vi "GUI.vi"() -> ()   [LabVIEW 2014]
uses:
  <vilib>/Platform/TimedLoop/XDataNode/timing_clust.ctl
  <vilib>/Platform/TimedLoop/XDataNode/nitl_modes.ctl
  <vilib>/Platform/TimedLoop/XDataNode/wakeup.ctl
  <vilib>/Instr/_visa.llb/VISA Configure Serial Port (Instr).vi
  <vilib>/platform/TimedLoop/XDataNode/XDataNode.xnode
  <vilib>/Platform/TimedLoop/XDataNode/XDNodeRunTimeDep.lvlib
panel:
  out "password is wrong":bool
  in  "write buffer":string
  in  "Write":bool
  in  "byte count":u32
  out "return count read":u32
  out "return count write":u32
  out "read buffer":string
  in  "Read":bool
  in  "timeout (10sec)":u32=10000
  in  "VISA resource name":refnum<visa-resource-name>
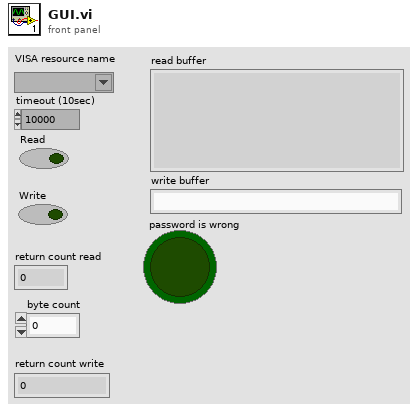
[diagram p1: front panel]
types:
  T1 = typedef "XDNodeRunTimeDep.lvlib/timing_clust.ctl" = cluster{"Expected End [f-1]":u64, "Actual End [f-1]":u64, "Finished Late? [f-1]":bool, "Expected End [i-1]":u64, "Actual End [i-1]":u64, "Finished Late? [i-1]":bool, "Expected Start [i]":u64, "Actual Start [i]":u64, "Expected Start [f]":u64, "Actual Start [f]":u64, "Source Name":string, "Structure Name":string, "Period":i64, "Deadline":i64, "Offset":i64, "Start":i64, "Priority":i32, "Timeout":i32, "Mode":T2, "Wakeup Reason":T3, "Error":errorcluster, "Source Type":string, "Secondary Source Type":string, "Global End Time":u64, "Global Start Time":u64, "Frame Duration":u64, "Iteration Duration":u64, "Assigned CPU":i32, "I/O Scan Engine Mode":u32}
  T2 = typedef "XDNodeRunTimeDep.lvlib/nitl_modes.ctl" = enum32{"No Change", "Process missed periods, maintain original phase", "Discard missed periods, maintain original phase", "Process missed periods, ignore original phase", "Discard missed periods, ignore original phase"}
  T3 = typedef "XDNodeRunTimeDep.lvlib/wakeup.ctl" = enum32{"Normal", "Aborted", "Asynchronous wakeup", "Timing source error", "Timed loop error", "Timeout"}
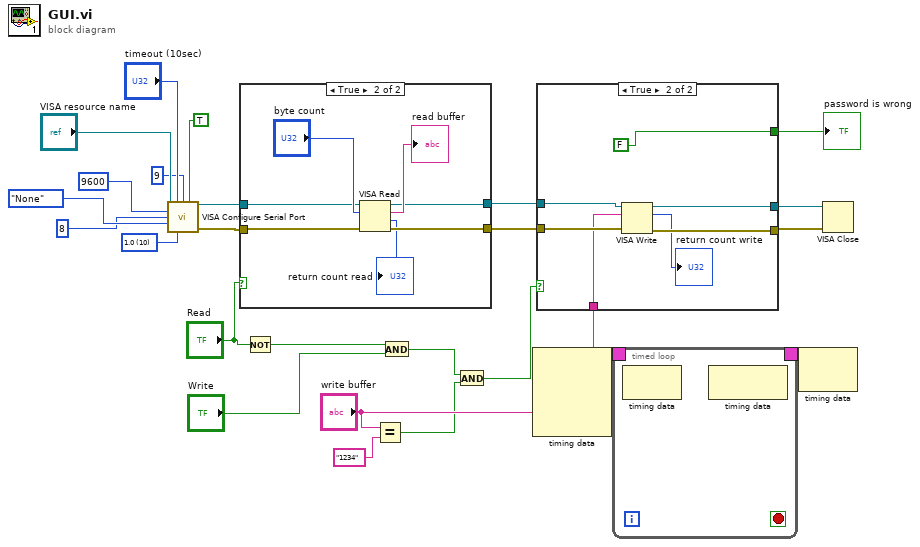
[diagram p0: block diagram]
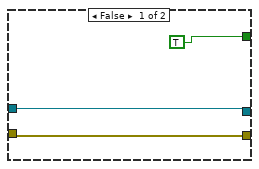
[diagram p3: hidden frame]
diagram:
  w22 = u16 10 items=["1.0"=10, "1.5"=15, "2.0"=20] ("stop bits (10: 1 bit)")
  n1 = call-poly "VISA Configure Serial Port"("VISA resource name"="VISA resource name", "timeout (10sec)"="timeout (10sec)", "termination char\n(0xA = '\\n' = LF)"=u8 9 ("termination char\n(0xA = '\\n' = LF)"), "Enable Termination\nChar (T)"=TRUE ("Enable Termination\nChar (T)"), "baud rate (9600)"=u32 9600, "data bits (8)"=u16 8, "parity (0:none)"=enum16{"None", "Odd", "Even", "Mark", "Space"}."None", "stop bits (10: 1 bit)"=w22) -> ("VISA resource name out"=w13:refnum<visa-resource-name>, "error out"=w11:errorcluster)  [unwired: 6 in]
  n2 = case shown="True" "Read" {
    tunnel: w11 -> [w27 w31]
    tunnel: [w26 w28] -> w12
    tunnel: [w27 w34] -> w10
    tunnel: w13 -> [w26 w29]
    frame False {
    }
    frame True {
      n3 = VISA Read(VISA resource name=w29, byte count="byte count", error in (no error)=w31) -> (VISA resource name out=w28:refnum<visa-resource-name>, read buffer=→"read buffer":string, return count=→"return count read":u32, error out=w34:errorcluster)
    }
  }
  n4 = Not(x="Read") -> (.not. x?=w16:bool)
  n5 = Equal?(x="write buffer", y="1234") -> (x = y?=w4:bool)
  n6 = And(x=w16, y="Write") -> (x .and. y?=w8:bool)
  n7 = And(x=w8, y=w4) -> (x .and. y?=w7:bool)
  n8 = node-c288() -> (w2:T1)  [unwired: 4 in]
  n9 = case shown="True" w7 {
    tunnel: w10 -> [w37 w44]
    tunnel: [w36 w43] -> w18
    tunnel: [w37 w42] -> w17
    tunnel: w12 -> [w36 w40]
    tunnel: "write buffer" -> [_ w39]
    tunnel: [TRUE FALSE] -> w5
    frame False {
    }
    frame True {
      n10 = VISA Write(VISA resource name=w40, write buffer=w39, error in (no error)=w44) -> (VISA resource name out=w43:refnum<visa-resource-name>, return count=→"return count write":u32, error out=w42:errorcluster)
    }
  }
  "password is wrong" <- w5
  n11 = timed-loop {
    timing: w2 -> [_]
    timing-out: [_] -> w1
    stop <- _ stop-if-true
    n12 = node-c288() -> ()  [unwired: 1 in, 1 out]
    n13 = node-c288() -> ()  [unwired: 1 in, 1 out]
  }
  n14 = node-c288(w1) -> ()  [unwired: 1 out]
  n15 = VISA Close(VISA resource name=w18, error in (no error)=w17) -> ()  [unwired: 1 out]
